vi "Cast to Interface.vi"(2 "Target Interface":refnum<class "IUnknown.lvclass">, 3 "Interfaceable Object":refnum<class "Interfaceable.lvclass">, 4 "error in (no error)":errorcluster) -> (0 "Concrete Interface":refnum<class "IUnknown.lvclass">, 1 "error out":errorcluster)   [LabVIEW 2009, in "Interfaceable.lvclass"]
doc: "Returns the concrete implementation of the given Interface for the interfaceable object. If the Interface is not found error 510201 is returned."
uses:
  Interfaceable.lvclass
  IUnknown Class/IUnknown.lvclass
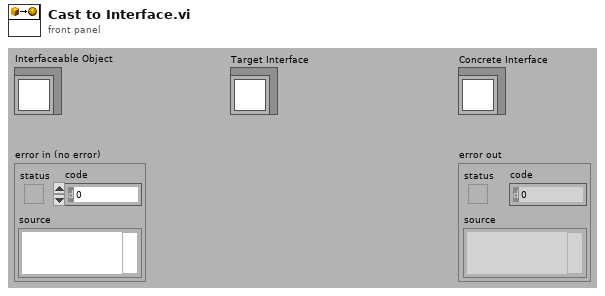
[diagram p1: front panel]
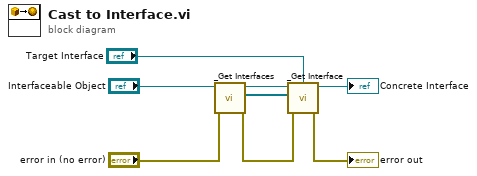
[diagram p0: block diagram]
diagram:
  n1 = call-dynamic "_Get Interfaces.vi"("error in (no error)"="error in (no error)", "Interfaceable in"="Interfaceable Object") -> ("error out"=w5:errorcluster, "Concrete Interfaces"=w2:refnum<class "IUnknown.lvclass">[], "Interfaceable out"=w7:refnum<class "Interfaceable.lvclass">)  [unwired: 7 in]
  n2 = call "_Get Interface.vi"("Desired Interface"="Target Interface", "Interfaceable in"=w7, "Available Concrete Interfaces"=w2, "error in (no error)"=w5) -> ("Concrete Interface"=→"Concrete Interface":refnum<class "IUnknown.lvclass">, "error out"=→"error out":errorcluster)  [unwired: 4 in]
